vi "Search Database To Get Member Info.vi"(8 "error in (no error)":errorcluster, 10 "searchContent":T1, 11 "userInfoManage in":refnum<class "UserInfoManageUI.lvclass">) -> (0 "error out":errorcluster, 2 "Result":string[][](array[string]), 3 "userInfoManage out":refnum<class "UserInfoManageUI.lvclass">)   [LabVIEW 2015, in "ActorManagement.lvlib" / "UserInfoManageUI.lvclass"]
uses:
  UserInfoManageUI.lvclass
  typedef/Member Search Condition(UI).ctl
  UserManagement/UserBasicInfo/UserBasicInfo.lvclass
  Plugin/Plugin.lvclass/Plugin.ctl
  PluginWithDatabase/PluginWithDatabase.lvclass/PluginWithDatabase.ctl
  DatabaseManagement/Database.lvclass
  UserManagement/Model/Model.lvclass
  Plugin/Plugin.lvclass
  PluginWithDatabase/PluginWithDatabase.lvclass
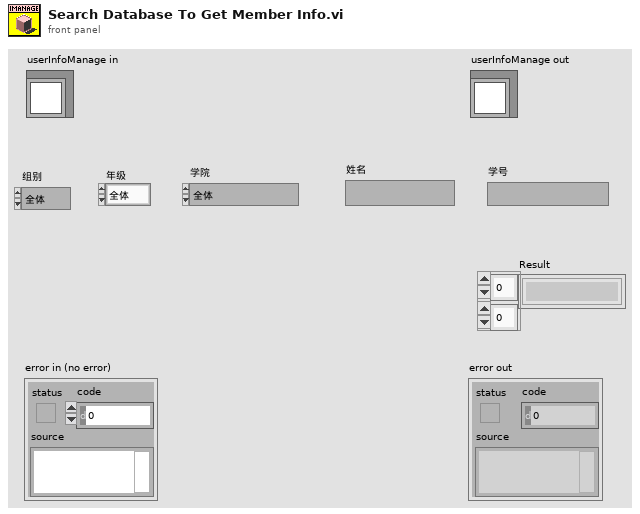
[diagram p1: front panel]
types:
  T1 = typedef "UserManagement.lvlib/UserBasicInfo.lvclass/Member Search Condition(UI).ctl" = cluster{"学号":string, "姓名":string, "学院":enum16{"全体", "机电工程学院", "电气工程学院", "航天学院", "能源学院", "理学院", "英才学院"}, "年级":enum16{"全体", "大二", "大三", "大四", "研一"}, "组别":enum16{"全体", "电控", "机械", "视觉"}}
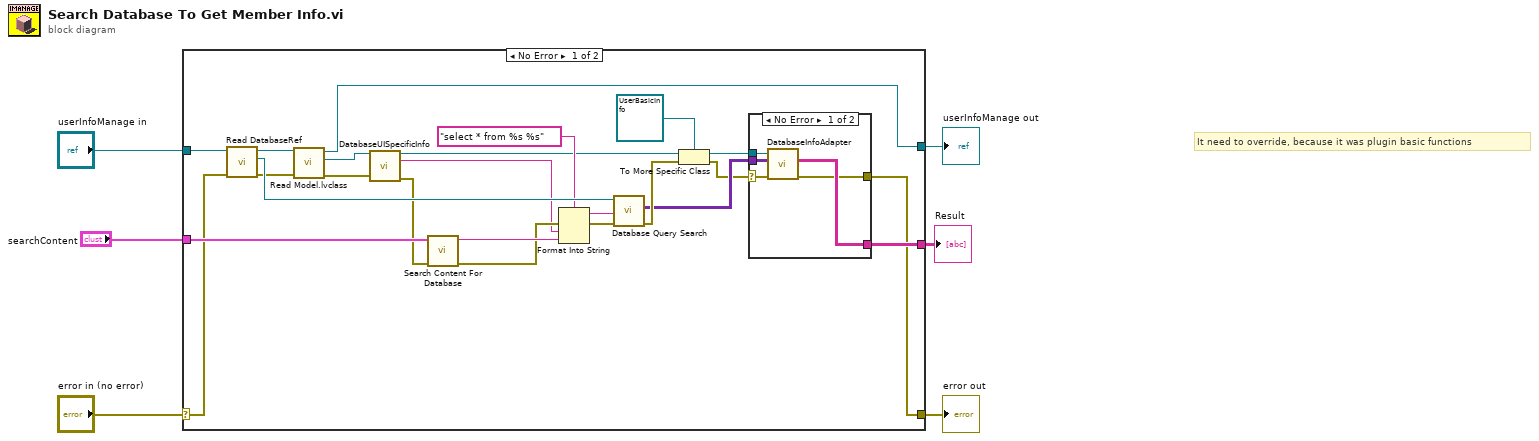
[diagram p0: block diagram]
diagram:
  # "It need to override, because it was plugin basic functions"
  n1 = case shown="No Error" "error in (no error)" {
    selector: "error in (no error)" -> [w29 w38]
    tunnel: [w7 w38] -> w5
    tunnel: [w8 w37] -> w3
    tunnel: "userInfoManage in" -> [w27 w37]
    tunnel: "searchContent" -> [w30 _]
    tunnel: [w9 _] -> w1
    frame No Error {
      n2 = call "Read DatabaseRef.vi"("error in (no error)"=w29, "Plugin in"=w27) -> ("error out"=w20:errorcluster, "Database.lvlib:Database"=w28:refnum<class "Database.lvclass">, "Plugin out"=w21:refnum<class "UserInfoManageUI.lvclass">)  [unwired: 7 in]
      n3 = call "Read Model.lvclass.vi"("error in (no error)"=w20, "PluginWithDatabase in"=w21) -> ("error out"=w18:errorcluster, "UserManagement.lvlib:Model"=w19:refnum<class "Model.lvclass">, "PluginWithDatabase out"=w8:refnum<class "UserInfoManageUI.lvclass">)  [unwired: 7 in]
      n4 = call-dynamic "DatabaseUISpecificInfo.vi"("Model.lvclass"=w19, "error in (no error)"=w18) -> ("Model.lvclass  out"=w15:refnum<class "Model.lvclass">, "TableName"=w16:string, "error out"=w17:errorcluster)  [unwired: 9 in, 2 out]
      n5 = call "Search Content For Database.vi"("error in (no error)"=w17, "searchContent"=w30) -> ("error out"=w24:errorcluster, "Query"=w25:string)  [unwired: 8 in]
      n6 = Format Into String(format string="select * from %s %s", error in=w24, w16, w25) -> (resulting string=w22:string, error out=w23:errorcluster)  [unwired: 1 in]
      n7 = call "Database Query Search.vi"("error in (no error)"=w23, "SQL query"=w22, "object in"=w28) -> ("error out"=w14:errorcluster, "recordset data"=w11:variant[][])  [unwired: 5 in, 2 out]
      n8 = To More Specific Class(target class=refnum<class "UserBasicInfo.lvclass"> refnum ("UserBasicInfo"), reference=w15, error in=w14) -> (specific class reference=w12:refnum<class "UserBasicInfo.lvclass">, error out=w10:errorcluster)
      n9 = case shown="No Error" w10 {
        selector: w10 -> [w33 w36]
        tunnel: w12 -> [w35 _]
        tunnel: w11 -> [w34 _]
        tunnel: [w32 _] -> w9
        tunnel: [w31 w36] -> w7
        frame No Error {
          n10 = call-dynamic "DatabaseInfoAdapter.vi"("error in (no error)"=w33, "recordset data"=w34, "UserBasicInfo"=w35) -> ("error out"=w31:errorcluster, "Result"=w32:string[][])  [unwired: 6 in, 1 out]
        }
        frame Error {
        }
      }
    }
    frame Error {
    }
  }
  "error out" <- w5
  "userInfoManage out" <- w3
  "Result" <- w1
